vi "Setup subWorkers.vi"(8 "error in":errorcluster, 11 "Container in":refnum<class "Container.lvclass">) -> (0 "error out":errorcluster, 3 "Container out":refnum<class "Container.lvclass">)   [LabVIEW 2023, in "Container.lvclass"]
doc: "<b>Note: Do not change the code in this VI!</b>\nThis VI performs a setup of all the statically-linked subWorkers that belong to the Worker that calls this VI. This VI is created automatically by the 'Create/Add Worker' tool and must be called <b>before</b> any statically linked subWorkers are called."
uses:
  Container.lvclass
  Container.lvclass/Container.ctl
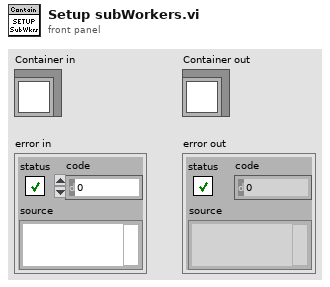
[diagram p1: front panel]
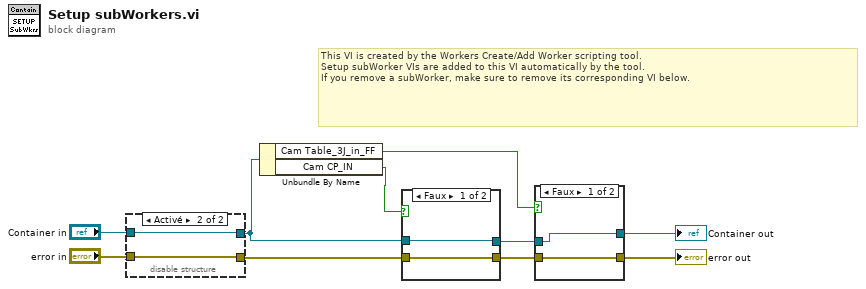
[diagram p0: block diagram]
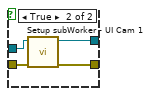
[diagram p2: hidden frame]
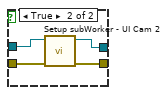
[diagram p3: hidden frame]
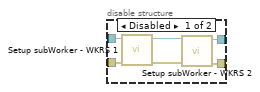
[diagram p4: hidden frame]
diagram:
  # "This VI is created by the Workers Create/Add Worker scripting tool.\nSetup subWorker VIs are added to this VI automatically by the tool.\nIf you remove a subWorker, make sure to remove its corresponding VI below."
  n1 = disable-structure shown="Activé" {
    disable-tunnel: "error in" -> [w16 w17]
    disable-tunnel: "Container in" -> [w15 w18]
    disable-tunnel: [w12 w17] -> w4
    disable-tunnel: [w11 w18] -> w1
    frame Disabled {
      n2 = call "Setup subWorker - WKRS 1.vi"("error in"=w16, "Container in"=w15) -> ("error out"=w13:errorcluster, "Container out"=w14:refnum<class "Container.lvclass">)  [unwired: 8 in]
      n3 = call "Setup subWorker - WKRS 2.vi"("error in"=w13, "Container in"=w14) -> ("error out"=w12:errorcluster, "Container out"=w11:refnum<class "Container.lvclass">)  [unwired: 8 in]
    }
    frame Enabled {
    }
  }
  n4 = Unbundle By Name(w1) -> ("Cam Table_3J_in_FF"=w6:bool, "Cam CP_IN"=w5:bool)
  n5 = case shown="Faux" w5 {
    tunnel: w4 -> [w19 w24]
    tunnel: [w19 w23] -> w3
    tunnel: [w20 w22] -> w2
    tunnel: w1 -> [w20 w21]
    frame False {
    }
    frame True {
      n6 = call "Setup subWorker - UI Cam 2.vi"("error in"=w24, "Container in"=w21) -> ("error out"=w23:errorcluster, "Container out"=w22:refnum<class "Container.lvclass">)  [unwired: 8 in]
    }
  }
  n7 = case shown="Faux" w6 {
    tunnel: [w25 w30] -> w8
    tunnel: [w26 w29] -> w7
    tunnel: w3 -> [w25 w28]
    tunnel: w2 -> [w26 w27]
    frame False {
    }
    frame True {
      n8 = call "Setup subWorker - UI Cam 1.vi"("error in"=w28, "Container in"=w27) -> ("error out"=w30:errorcluster, "Container out"=w29:refnum<class "Container.lvclass">)  [unwired: 8 in]
    }
  }
  "error out" <- w8
  "Container out" <- w7
